vi "Galvo preview code.vi"() -> ()   [LabVIEW 2024]
uses:
  <vilib>/DAQmx/write.llb/DAQmx Write (Analog 2D DBL NChan NSamp).vi
  <vilib>/DAQmx/create/channels.llb/DAQmx Create Channel (AO-Voltage-Basic).vi
  <vilib>/DAQmx/miscellaneous.llb/DAQmx Fill In Error Info.vi
  <vilib>/measure/NI_MABase.lvlib
panel:
  in  "stop":bool
  in  "offset 2":dbl format="%0.2p"
  in  "phase 2":dbl format="%.2p"
  in  "amplitude 2":dbl=1.0 format="%0.2p"
  in  "phase":dbl format="%.2p"
  in  "amplitude":dbl=1.0 format="%0.2p"
  in  "offset":dbl format="%0.2p"
  out "Waveform Chart 2":waveform(dbl)(graph)
  out "Waveform Chart":waveform(dbl)(graph)
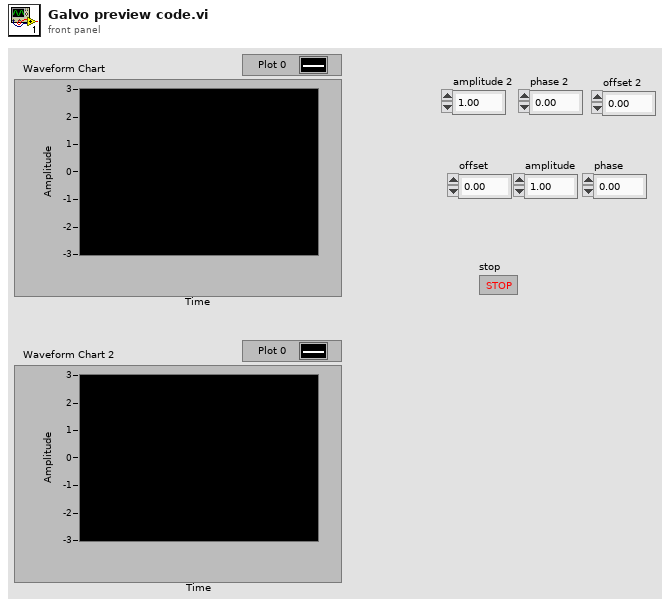
[diagram p1: front panel]
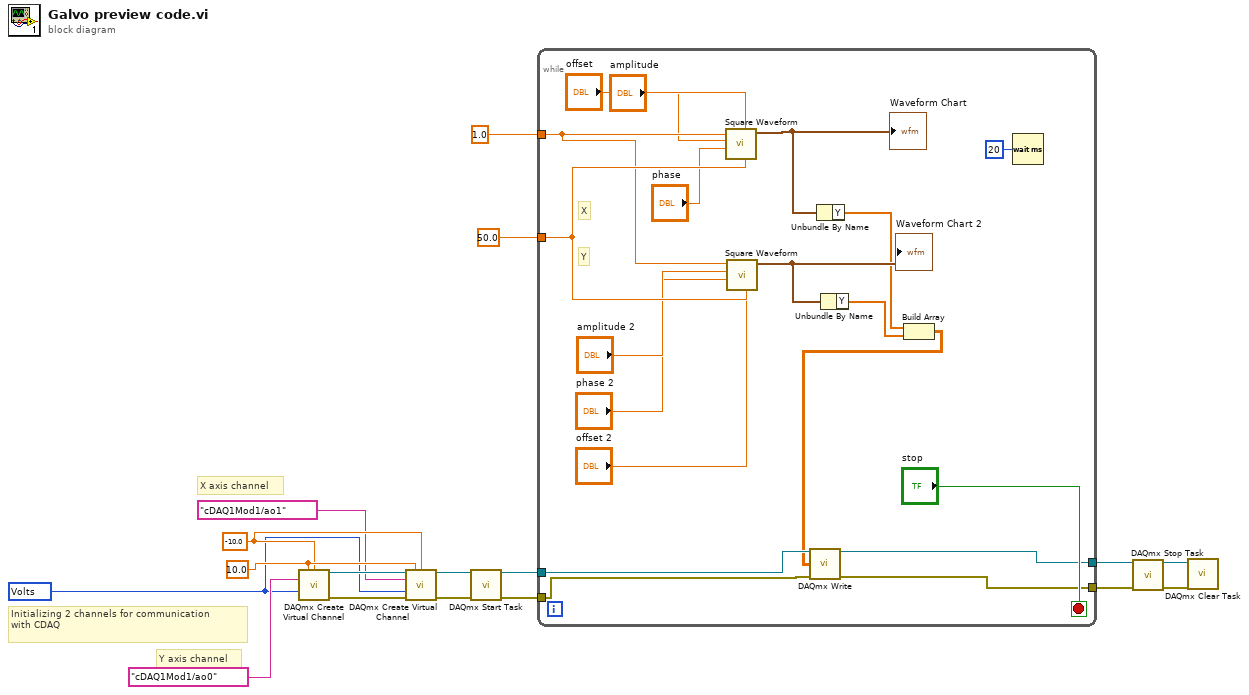
[diagram p0: block diagram]
diagram:
  w9 = 10348 items=["Volts"=10348, "From Custom Scale"=10065] ("units")
  w13 = 10.0 ("maximum value")
  w12 = -10.0 ("minimum value")
  # "Initializing 2 channels for communication\nwith CDAQ"
  # "X axis channel"
  # "Y axis channel"
  n1 = call-poly <vilib>:"DAQmx Create Virtual Channel.vi"("maximum value"=w13, "minimum value"=w12, "physical channels"=tag "cDAQ1Mod1/ao0", "units"=w9) -> ("task out"=w15:refnum<k21>, "error out"=w14:errorcluster)  [unwired: 10 in]
  n2 = call-poly <vilib>:"DAQmx Create Virtual Channel.vi"("task in"=w15, "maximum value"=w13, "minimum value"=w12, "physical channels"=tag "cDAQ1Mod1/ao1", "units"=w9, "error in"=w14) -> ("task out"=w8:refnum<k21>, "error out"=w7:errorcluster)  [unwired: 8 in]
  n3 = call <vilib>:"DAQmx Start Task.vi"("task/channels in"=w8, "error in"=w7) -> ("task out"=w6:refnum<k21>, "error out"=w5:errorcluster)  [unwired: 12 in]
  n4 = while {
    tunnel: 50.0 ("duty cycle (%)") -> [w36]
    tunnel: 1.0 ("frequency") -> [w35]
    tunnel: w6 -> [w26]
    tunnel: w5 -> [w25]
    tunnel: [w19] -> w2
    tunnel: [w18] -> w1
    stop <- "stop" stop-if-true
    # "Y"
    # "X"
    n5 = call <vilib>:"Square Waveform.vi"("duty cycle (%)"=w36, "offset"="offset", "phase"="phase", "amplitude"="amplitude", "frequency"=w35) -> ("signal out"=w23:waveform(dbl))  [unwired: 5 in, 1 out]
    "Waveform Chart" <- w23
    n6 = call <vilib>:"Square Waveform.vi"("duty cycle (%)"=w36, "offset"="offset 2", "phase"="phase 2", "amplitude"="amplitude 2", "frequency"=w35) -> ("signal out"=w24:waveform(dbl))  [unwired: 5 in, 1 out]
    "Waveform Chart 2" <- w24
    n7 = Unbundle By Name(w23) -> ("Y"=w22:dbl[])
    n8 = Unbundle By Name(w24) -> ("Y"=w21:dbl[])
    n9 = Build Array(w22, w21) -> (w20:dbl[][])
    n10 = call-poly <vilib>:"DAQmx Write.vi"("task/channels in"=w26, "data"=w20, "error in"=w25) -> ("task out"=w19:refnum<k21>, "error out"=w18:errorcluster)  [unwired: 10 in, 1 out]
    n11 = Wait (ms)(milliseconds to wait=u32 20) -> ()  [unwired: 1 out]
  }
  n12 = call <vilib>:"DAQmx Stop Task.vi"("task/channels in"=w2, "error in"=w1) -> ("task out"=w4:refnum<k21>, "error out"=w3:errorcluster)  [unwired: 12 in]
  n13 = call <vilib>:"DAQmx Clear Task.vi"("task in"=w4, "error in"=w3) -> ()  [unwired: 13 in, 1 out]
